vi "LabVIEW_VNA_ESP.vi"() -> ()   [LabVIEW 2020]
uses:
  <vilib>/Analysis/Matrix/Numeric/Conversions/Array To Matrix - RA.vi
  <vilib>/Analysis/Matrix/NI_Matrix.lvlib
panel:
  in  "Entrées pour la fonction Plot":T1={"Chemin du fichiers de mesures (doit contenir le nom du fichier)"=path "", "Type de mesure"="1", "Chemin du fichier parametres (doit contenir le nom du fichier)"=path "", "pas"="", "Coordonnée du point d'arrivée "="", "Coordonnée du point de départ "=""}
  out "Scan 2D mag S12 2":dbl[][](graph)
  out "Scan 2D phase S12 2":dbl[][](graph)
  out "Scan 2D mag S21 2":dbl[][](graph)
  out "Scan 2D phase S21 2":dbl[][](graph)
  out "Rotation mag S21 3":cluster{dbl[], dbl[]}(graph)
  out "Rotation phase S12 2":cluster{dbl[], dbl[]}(graph)
  out "Rotation mag S21 2":cluster{dbl[], dbl[]}(graph)
  out "Rotation phase S21 2":cluster{dbl[], dbl[]}(graph)
  in  "?":bool
  in  "Chemins":cluster{"script python":path, "save path":path}={"script python"=path "C:/Users/Thomas/Documents/Galaad_B/labview/VNA_ESP_10_06_25.py", "save path"=path "C:/Users/Thomas/Documents/Galaad_B/vna_data_test_galaad"}
  in  "IP":T2={"IP VNA"="GPIB0::16::INSTR", "IP ESP Scan 2D"="GPIB0::1::INSTR", "IP ESP Rotation"="GPIB0::2::INSTR"}
  in  "Paramètres de mesures (rotation et balayage)":T3={"Axe"="5", "unité"="2", "coordonnées du point d'arrivé"="10", "coordonnées du point de départ"="0", "pas"="1", "moyennage sur x mesures"="20", "limite basse du balayage en fréquence (GHz)"="110", "limite haute du balayage en fréquence (GHz)"="170", "nombre de points entre les deux limites de fréquences"="201", "IFBW (Hz)"="1000", "band"="WR6.5_Galaad.csa", "sens (aucun effet sur la fonction balayage)"="-to+", "fréquence pour les plots (GHz)"="140", "Nom du fichier"=""}
  in  "Entrées pour la fonction Move":T4={"Axes"="1", "mouvement"="5", "absolu / relatif"="1", "vitesse"="1", "unité"="2", "ESP"=""}
  out "Scan 2D phase S21":dbl[][](graph)
  out "Scan 2D mag S21":dbl[][](graph)
  out "Scan 2D phase S12":dbl[][](graph)
  out "Rotation mag S21":cluster{dbl[], dbl[]}(graph)
  out "Rotation phase S21":cluster{dbl[], dbl[]}(graph)
  out "Rotation phase S12":cluster{dbl[], dbl[]}(graph)
  out "Rotation mag S21":cluster{dbl[], dbl[]}(graph)
  out "Scan 2D mag S12":dbl[][](graph)
  in  "Operation":string(combo)="Balayage_2D_VNA_ESP"
  out "error out":errorcluster caption="sortie d'erreur"
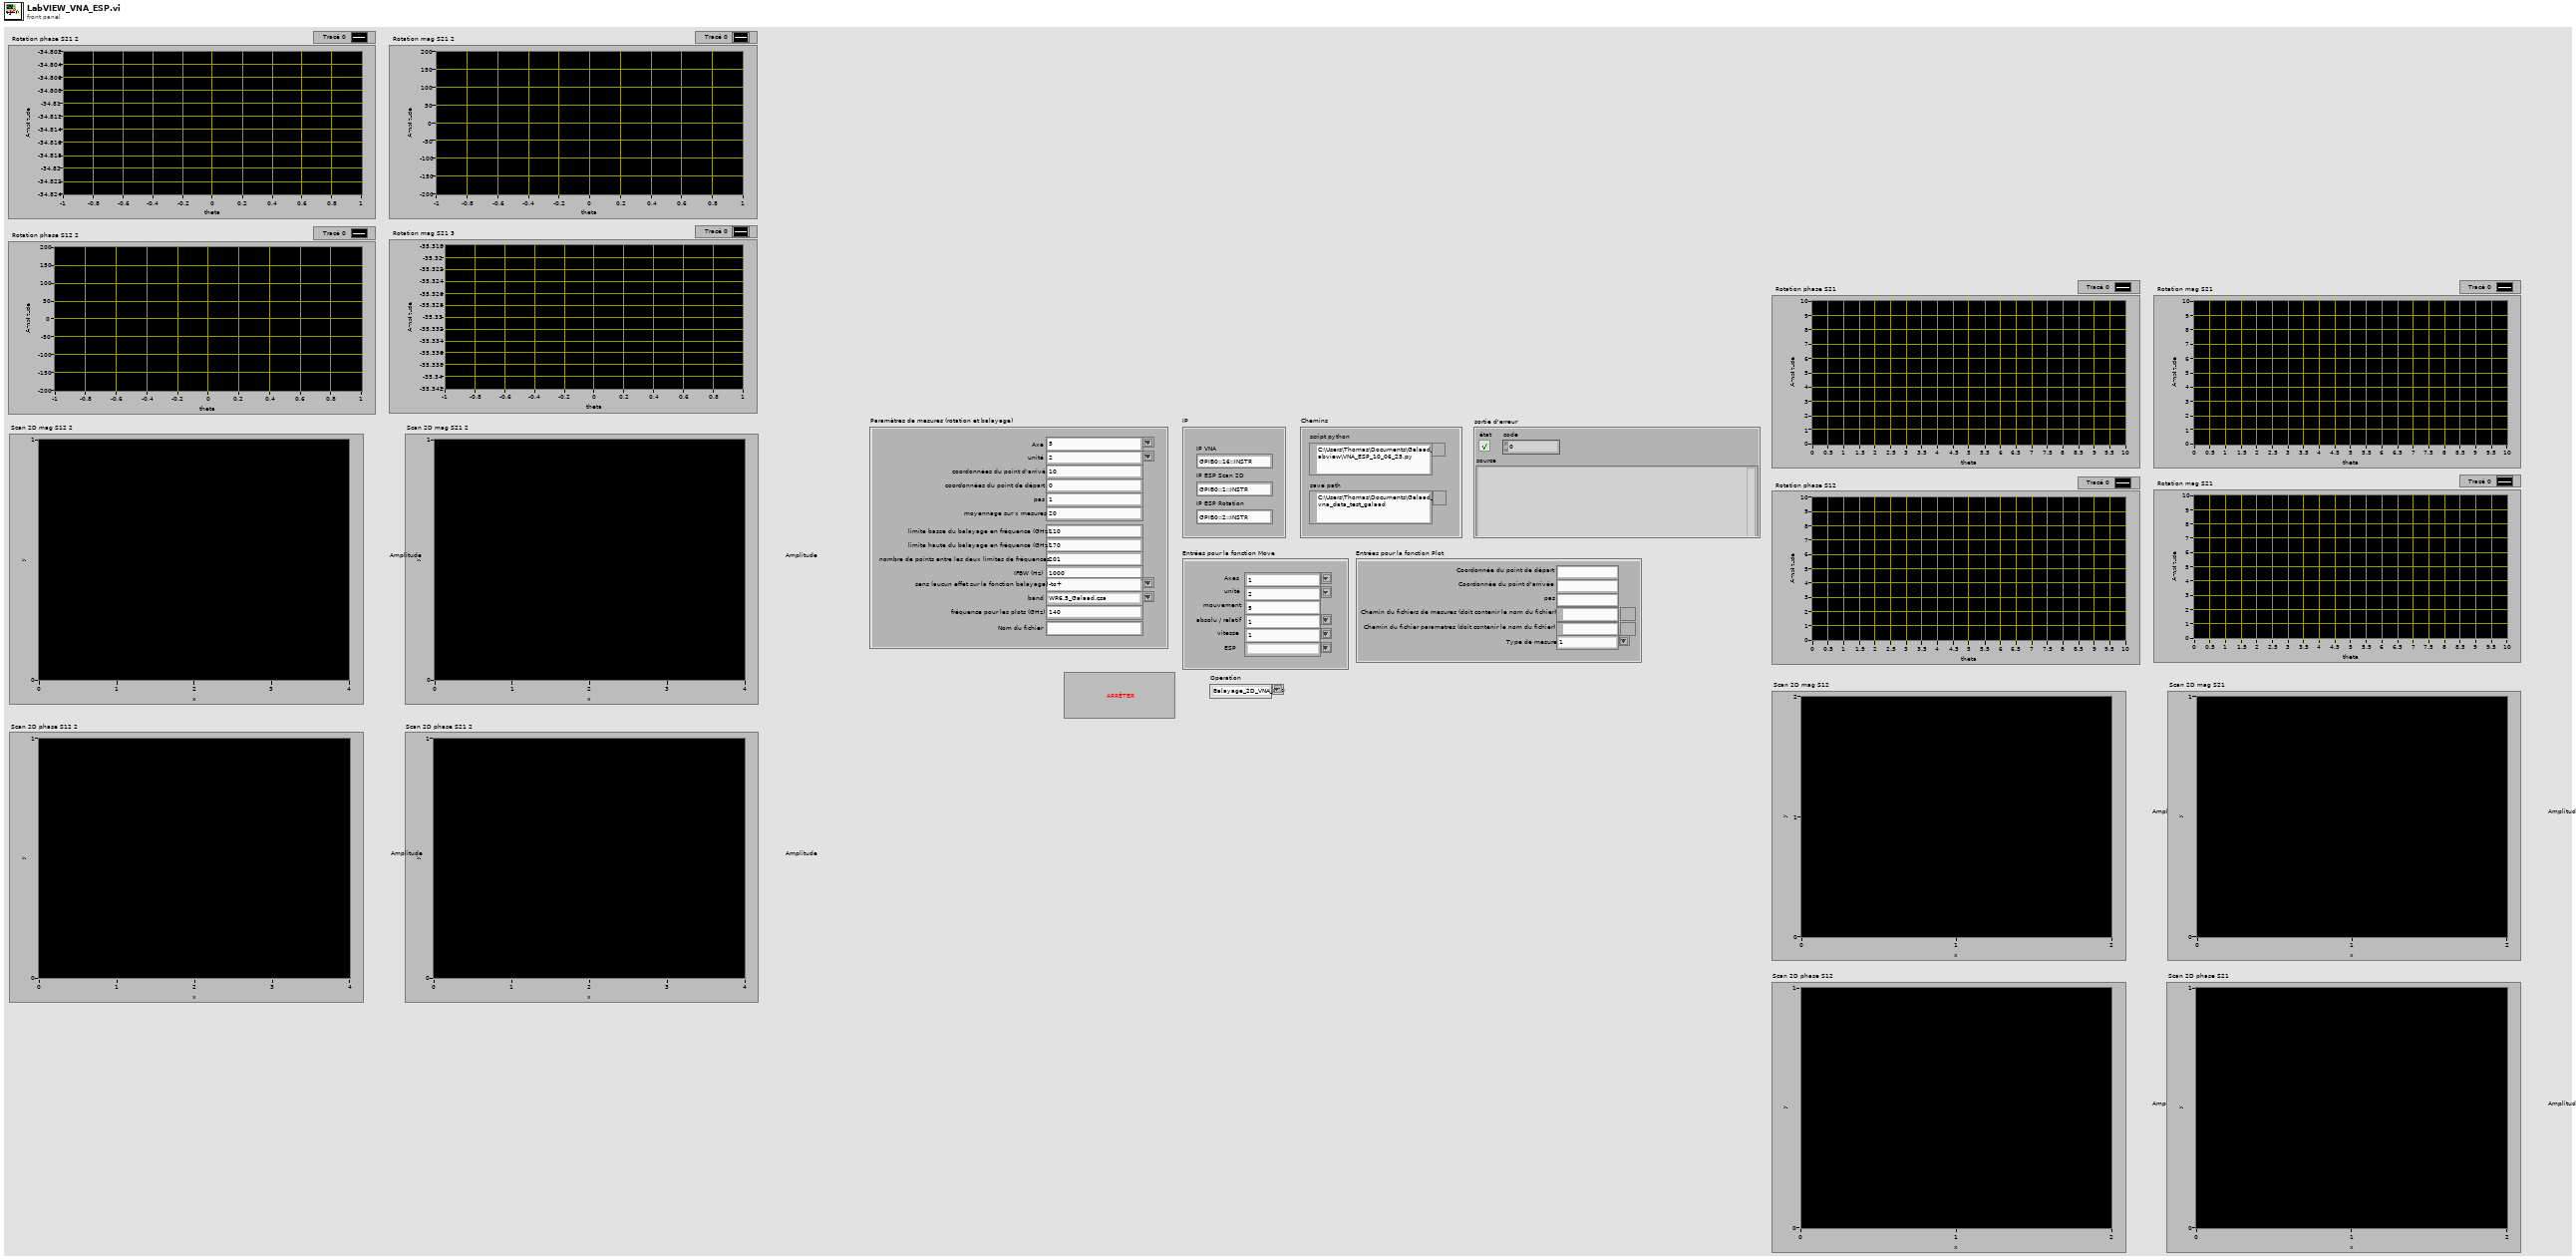
[diagram p1: front panel]
types:
  T1 = cluster{"Chemin du fichiers de mesures (doit contenir le nom du fichier)":path, "Type de mesure":string, "Chemin du fichier parametres (doit contenir le nom du fichier)":path, "pas":string, "Coordonnée du point d'arrivée ":string, "Coordonnée du point de départ ":string}
  T2 = cluster{"IP VNA":string, "IP ESP Scan 2D":string, "IP ESP Rotation":string}
  T3 = cluster{"Axe":string, "unité":string, "coordonnées du point d'arrivé":string, "coordonnées du point de départ":string, "pas":string, "moyennage sur x mesures":string, "limite basse du balayage en fréquence (GHz)":string, "limite haute du balayage en fréquence (GHz)":string, "nombre de points entre les deux limites de fréquences":string, "IFBW (Hz)":string, "band":string, "sens (aucun effet sur la fonction balayage)":string, "fréquence pour les plots (GHz)":string, "Nom du fichier":string}
  T4 = cluster{"Axes":string, "mouvement":string, "absolu / relatif":string, "vitesse":string, "unité":string, "ESP":string}
  T5 = cluster{"Axe":string, "unité":string, "coordonnées du point d'arrivé":string, "coordonnées du point de départ":string, "pas":string, "moyennage sur x mesures":string, "limite basse du balayage en fréquence (GHz)":string, "limite haute du balayage en fréquence (GHz)":string, "nombre de points entre les deux limites de fréquences":string, "IFBW (Hz)":string, "band":string, "IP VNA":string, "IP ESP Scan 2D":string, string, "fréquence pour les plots (GHz)":string, "Nom du fichier":string}
  T6 = cluster{"Axe":string, "unité":string, "coordonnées du point d'arrivé":string, "coordonnées du point de départ":string, "pas":string, "moyennage sur x mesures":string, "limite basse du balayage en fréquence (GHz)":string, "limite haute du balayage en fréquence (GHz)":string, "nombre de points entre les deux limites de fréquences":string, "IFBW (Hz)":string, "band":string, "sens (aucun effet sur la fonction balayage)":string, "fréquence pour les plots (GHz)":string, "IP VNA":string, "IP ESP Rotation":string, string, "Nom du fichier":string}
  T7 = cluster{"Axes":string, "unité":string, "mouvement":string, "absolu / relatif":string, "vitesse":string, "IP ESP Rotation":string}
  T8 = cluster{"Axes":string, "unité":string, "mouvement":string, "absolu / relatif":string, "vitesse":string, "IP ESP Scan 2D":string}
  T9 = typedef "NI_Matrix.lvlib/RealMatrix.ctl" = dbl[][]
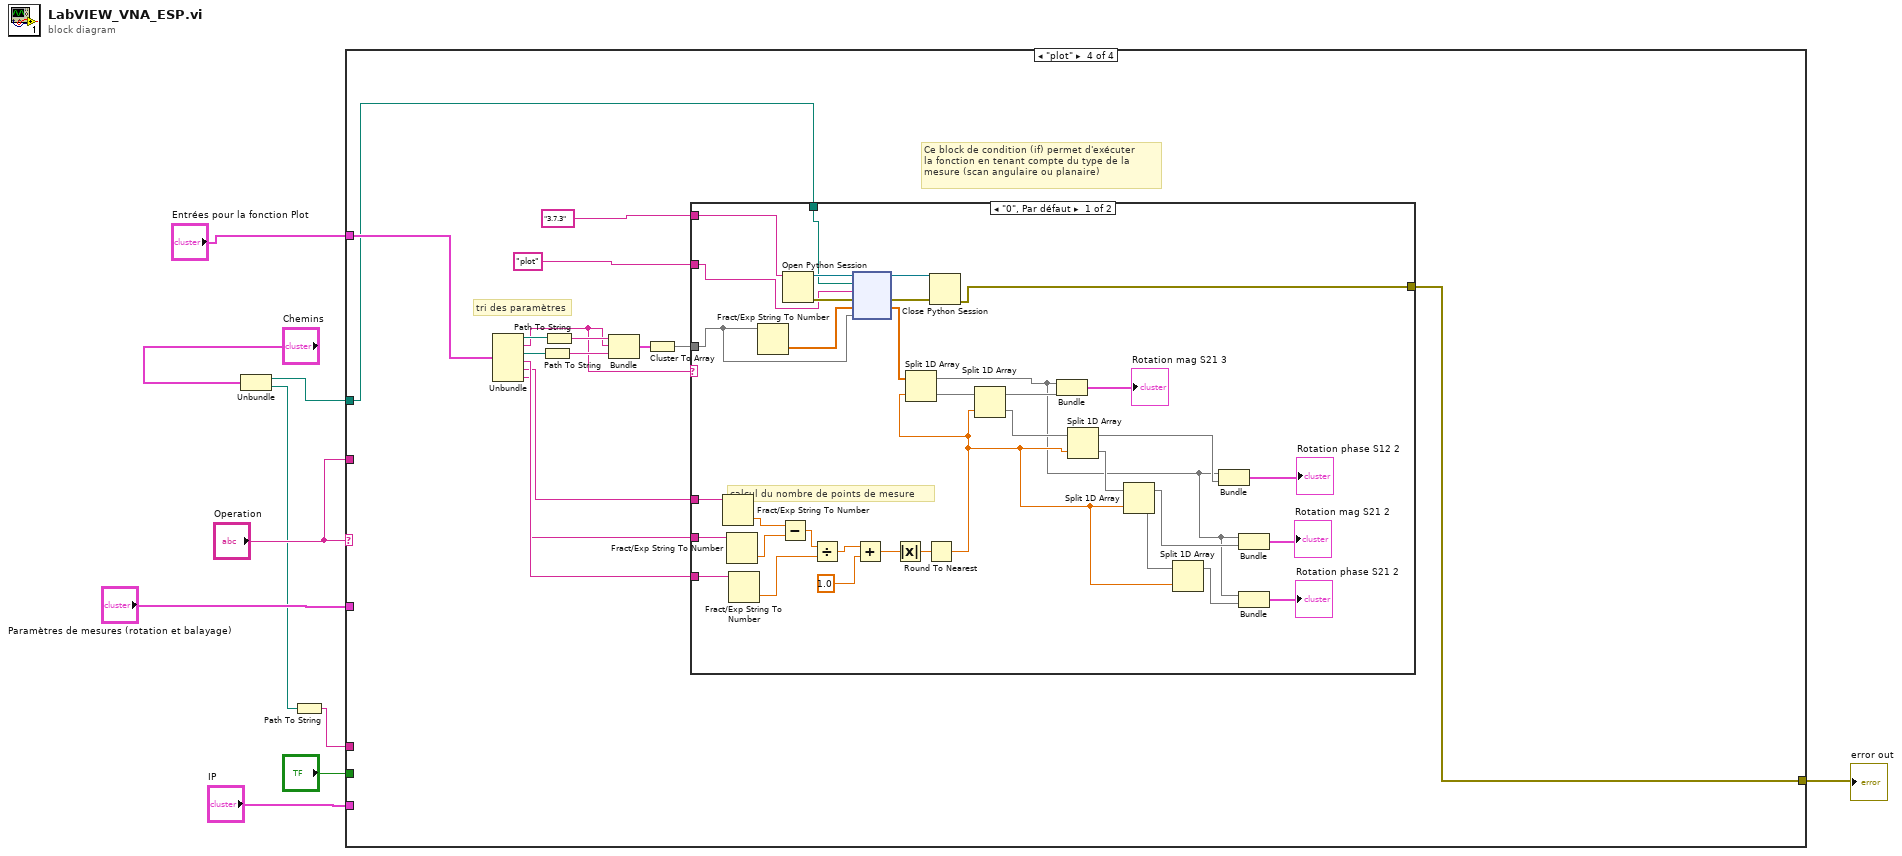
[diagram p0: block diagram]
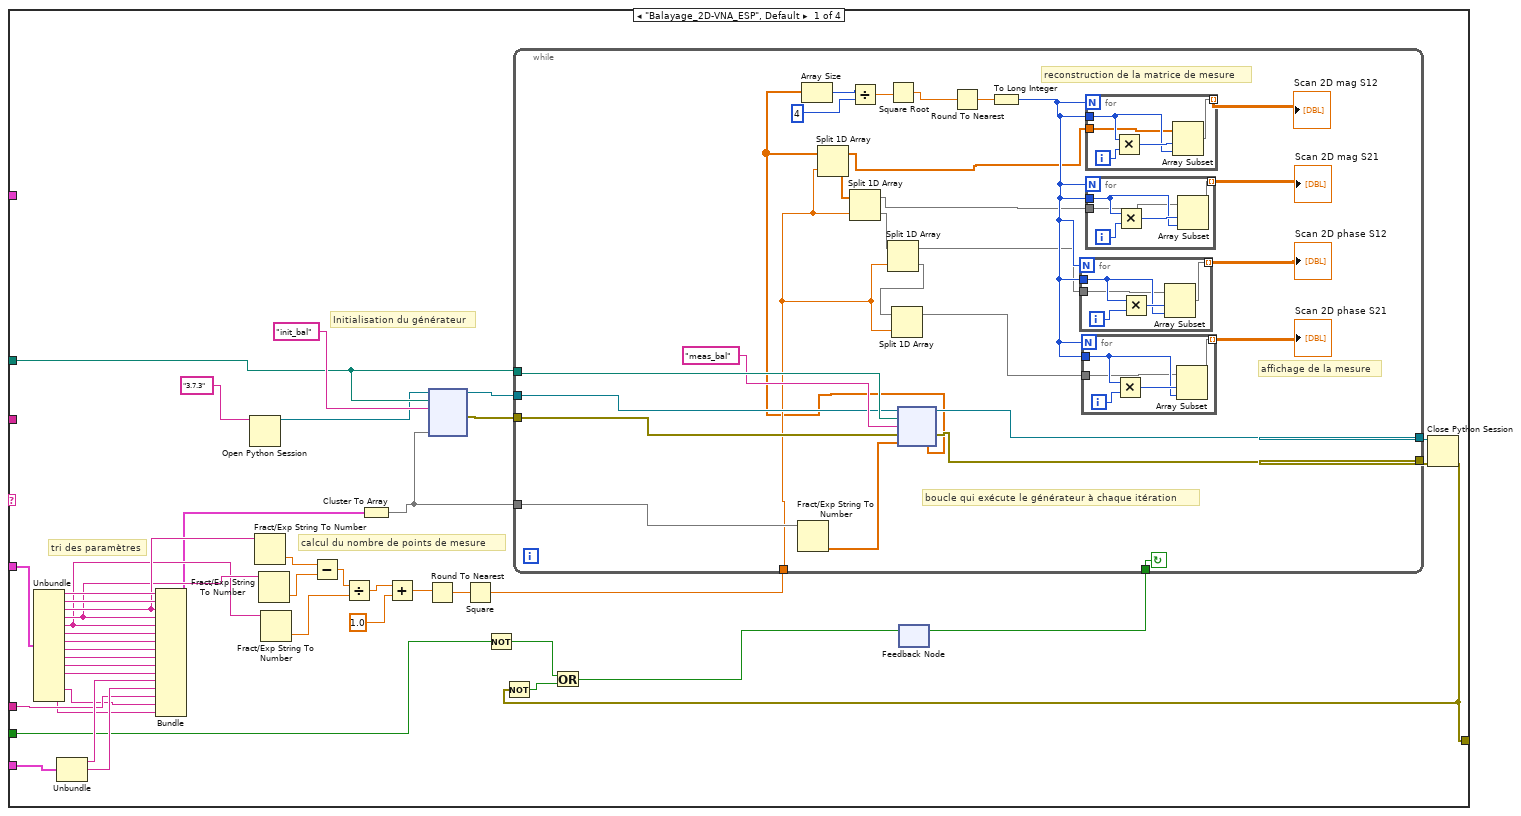
[diagram p2: hidden frame]
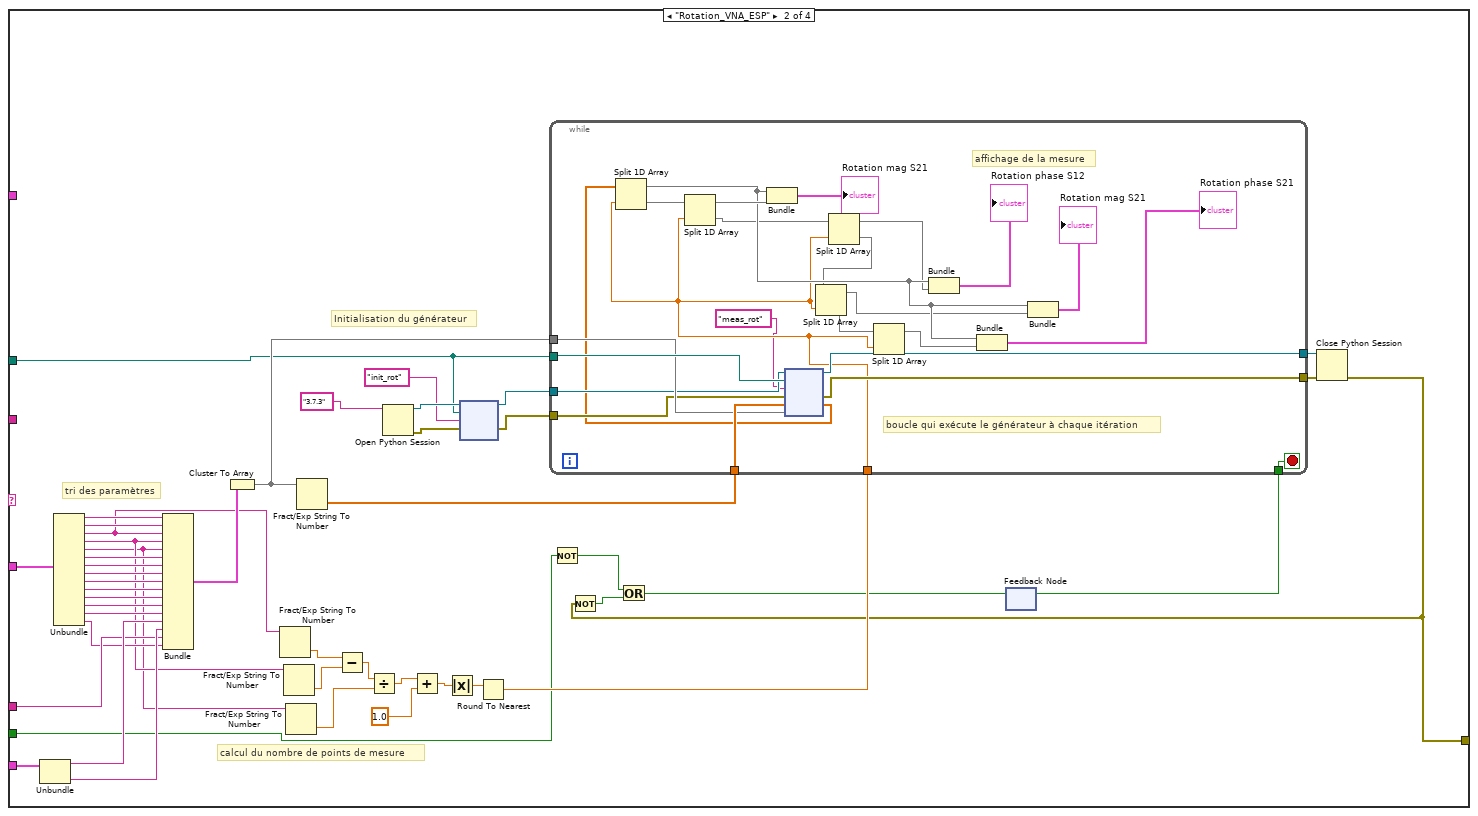
[diagram p3: hidden frame]
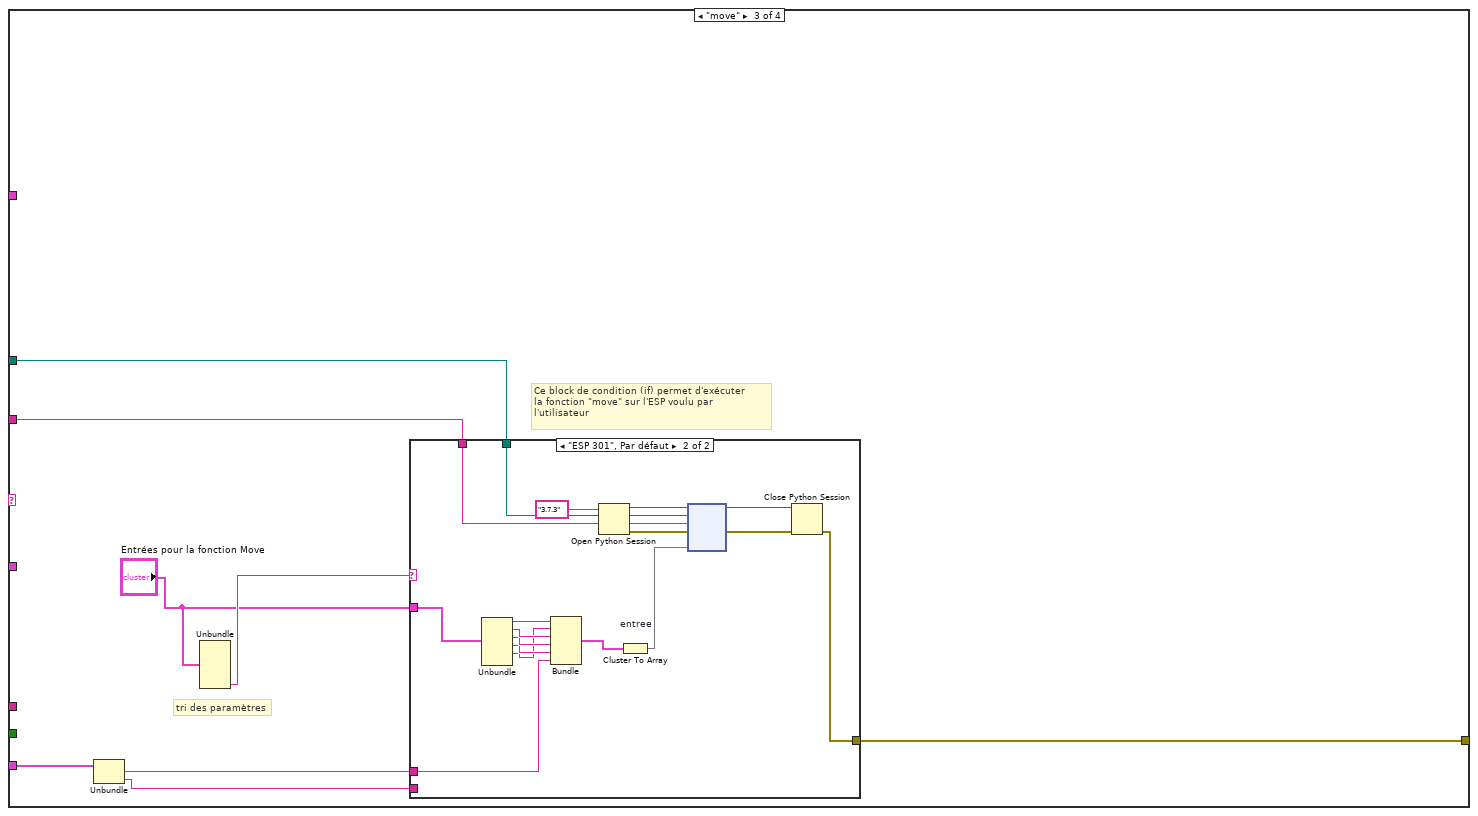
[diagram p4: hidden frame]
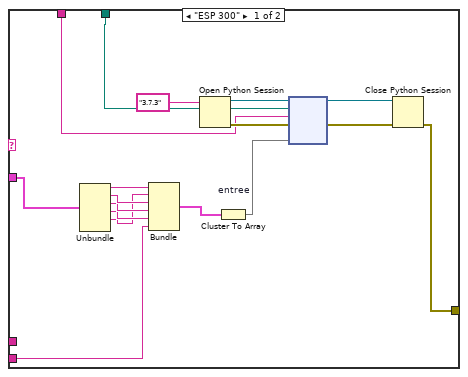
[diagram p5: hidden frame]
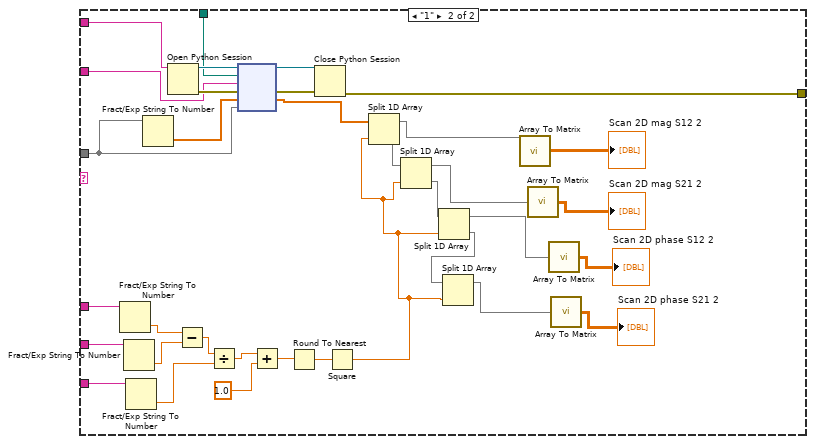
[diagram p6: hidden frame]
diagram:
  n1 = Unbundle("Chemins") -> ("script python"=w4:path, "save path"=w3:path)
  n2 = Path To String(path=w3) -> (string=w10:string)
  n3 = case shown="\"plot\"" "Operation" {
    tunnel: w10 -> [w31 w124 _ _]
    tunnel: "Paramètres de mesures (rotation et balayage)" -> [w34 w139 _ _]
    tunnel: "IP" -> [w46 w138 w177 _]
    tunnel: w4 -> [w19 w114 w174 w215]
    tunnel: [w12 w104 w173 w214] -> w7
    tunnel: "Operation" -> [_ _ w172 _]
    tunnel: "?" -> [w27 w105 _ _]
    tunnel: "Entrées pour la fonction Plot" -> [_ _ _ w216]
    frame "Balayage_2D-VNA_ESP", Default {
      # "tri des paramètres"
      # "calcul du nombre de points de mesure"
      # "Initialisation du générateur"
      n4 = Unbundle(w34) -> ("Axe"=w45:string, "unité"=w44:string, "coordonnées du point d'arrivé"=w37:string, "coordonnées du point de départ"=w36:string, "pas"=w35:string, "moyennage sur x mesures"=w43:string, "limite basse du balayage en fréquence (GHz)"=w42:string, "limite haute du balayage en fréquence (GHz)"=w41:string, "nombre de points entre les deux limites de fréquences"=w40:string, "IFBW (Hz)"=w39:string, "band"=w38:string, "fréquence pour les plots (GHz)"=w30:string, "Nom du fichier"=w29:string)  [unwired: 1 out]
      n5 = Unbundle(w46) -> ("IP VNA"=w33:string, "IP ESP Scan 2D"=w32:string)  [unwired: 1 out]
      n6 = Bundle("Axe"=w45, "unité"=w44, "coordonnées du point d'arrivé"=w37, "coordonnées du point de départ"=w36, "pas"=w35, "moyennage sur x mesures"=w43, "limite basse du balayage en fréquence (GHz)"=w42, "limite haute du balayage en fréquence (GHz)"=w41, "nombre de points entre les deux limites de fréquences"=w40, "IFBW (Hz)"=w39, "band"=w38, "IP VNA"=w33, "IP ESP Scan 2D"=w32, w31, "fréquence pour les plots (GHz)"=w30, "Nom du fichier"=w29) -> (w17:T5)  [unwired: 1 in]
      n7 = Open Python Session(python version="3.7.3") -> (session out=w18:refnum<k35>)  [unwired: 2 in, 1 out]
      n8 = Fract/Exp String To Number(string=w37) -> (number=w51:dbl)  [unwired: 3 in, 1 out]
      n9 = Fract/Exp String To Number(string=w36) -> (number=w52:dbl)  [unwired: 3 in, 1 out]
      n10 = Fract/Exp String To Number(string=w35) -> (number=w53:dbl)  [unwired: 3 in, 1 out]
      n11 = Subtract(x=w51, y=w52) -> (x-y=w48:dbl)
      n12 = Divide(x=w48, y=w53) -> (x/y=w49:dbl)
      n13 = Cluster To Array(cluster=w17) -> (array=w16:string[])
      n14 = Add(x=w49, y=1.0) -> (x+y=w50:dbl)
      n15 = Round To Nearest(number=w50) -> (nearest integer value=w28:dbl)
      n16 = node(w18, w19, "init_bal", w16) -> (w21:refnum<k35>, w15:errorcluster)  [unwired: 4 in, 2 out]
      n17 = Square(x=w28) -> (x^2=w11:dbl)
      n18 = Not(x=w27) -> (.not. x?=w26:bool)
      n19 = feedback #1() -> (w23:bool)  [unwired: 1 in]
      n20 = while {
        tunnel: w23 -> [w81]
        tunnel: w19 -> [w80]
        tunnel: w21 -> [w77]
        tunnel: w16 -> [w76]
        tunnel: w15 -> [w75]
        tunnel: [w74] -> w14
        tunnel: [w73] -> w13
        tunnel: w11 -> [w56]
        stop <- w81 continue-if-true
        # "affichage de la mesure"
        # "reconstruction de la matrice de mesure"
        # "boucle qui exécute le générateur à chaque itération"
        n21 = Fract/Exp String To Number(string=w76) -> (number=w79:dbl[])  [unwired: 3 in, 1 out]
        n22 = node(w77, w80, "meas_bal", w75, w79) -> (w74:refnum<k35>, w73:errorcluster, w54:dbl[])  [unwired: 2 out]
        n23 = Array Size(array=w54) -> (size(s)=w63:i32)
        n24 = Split 1D Array(array=w54, index=w56) -> (first subarray=w55:dbl[], second subarray=w60:dbl[])
        n25 = Divide(x=w63, y=4) -> (x/y=w64:dbl)
        n26 = Split 1D Array(array=w60, index=w56) -> (first subarray=w69:dbl[], second subarray=w59:dbl[])
        n27 = Square Root(x=w64) -> (sqrt(x)=w61:dbl)
        n28 = Split 1D Array(array=w59, index=w56) -> (first subarray=w70:dbl[], second subarray=w58:dbl[])
        n29 = Split 1D Array(array=w58, index=w56) -> (first subarray=w71:dbl[])  [unwired: 1 out]
        n30 = Round To Nearest(number=w61) -> (nearest integer value=w62:dbl)
        n31 = To Long Integer(number=w62) -> (32bit integer=w72:i32)
        n32 = for {
          N: w72 -> [_]
          tunnel: [w91] -> w67 mode=indexing
          tunnel: w72 -> [w88]
          tunnel: w70 -> [w87]
          i -> [w90]
          n33 = Multiply(x=w88, y=w90) -> (x*y=w89:i32)
          n34 = Array Subset(array=w87, index=w89, length=w88) -> (w91:dbl[])
        }
        "Scan 2D phase S12" <- w67
        n35 = for {
          N: w72 -> [_]
          tunnel: [w86] -> w68 mode=indexing
          tunnel: w72 -> [w83]
          tunnel: w71 -> [w82]
          i -> [w85]
          n36 = Multiply(x=w83, y=w85) -> (x*y=w84:i32)
          n37 = Array Subset(array=w82, index=w84, length=w83) -> (w86:dbl[])
        }
        "Scan 2D phase S21" <- w68
        n38 = for {
          N: w72 -> [_]
          tunnel: [w101] -> w65 mode=indexing
          tunnel: w72 -> [w98]
          tunnel: w55 -> [w97]
          i -> [w100]
          n39 = Multiply(x=w98, y=w100) -> (x*y=w99:i32)
          n40 = Array Subset(array=w97, index=w99, length=w98) -> (w101:dbl[])
        }
        "Scan 2D mag S12" <- w65
        n41 = for {
          N: w72 -> [_]
          tunnel: [w96] -> w66 mode=indexing
          tunnel: w72 -> [w93]
          tunnel: w69 -> [w92]
          i -> [w95]
          n42 = Multiply(x=w93, y=w95) -> (x*y=w94:i32)
          n43 = Array Subset(array=w92, index=w94, length=w93) -> (w96:dbl[])
        }
        "Scan 2D mag S21" <- w66
      }
      n44 = Close Python Session(session in=w14, error in=w13) -> (11:w12:errorcluster)
      n45 = Not(x=w12) -> (.not. x?=w25:bool)
      n46 = Or(x=w26, y=w25) -> (x .or. y?=w24:bool)
      n47 = feedback-in #1(w24) -> ()
    }
    frame "Rotation_VNA_ESP" {
      # "calcul du nombre de points de mesure"
      # "Initialisation du générateur"
      # "tri des paramètres"
      n48 = Unbundle(w138) -> ("IP VNA"=w126:string, "IP ESP Rotation"=w125:string)  [unwired: 1 out]
      n49 = Unbundle(w139) -> ("Axe"=w136:string, "unité"=w135:string, "coordonnées du point d'arrivé"=w122:string, "coordonnées du point de départ"=w121:string, "pas"=w120:string, "moyennage sur x mesures"=w134:string, "limite basse du balayage en fréquence (GHz)"=w133:string, "limite haute du balayage en fréquence (GHz)"=w132:string, "nombre de points entre les deux limites de fréquences"=w131:string, "IFBW (Hz)"=w130:string, "band"=w129:string, "sens (aucun effet sur la fonction balayage)"=w128:string, "fréquence pour les plots (GHz)"=w127:string, "Nom du fichier"=w123:string)
      n50 = Bundle("Axe"=w136, "unité"=w135, "coordonnées du point d'arrivé"=w122, "coordonnées du point de départ"=w121, "pas"=w120, "moyennage sur x mesures"=w134, "limite basse du balayage en fréquence (GHz)"=w133, "limite haute du balayage en fréquence (GHz)"=w132, "nombre de points entre les deux limites de fréquences"=w131, "IFBW (Hz)"=w130, "band"=w129, "sens (aucun effet sur la fonction balayage)"=w128, "fréquence pour les plots (GHz)"=w127, "IP VNA"=w126, "IP ESP Rotation"=w125, w124, "Nom du fichier"=w123) -> (w137:T6)  [unwired: 1 in]
      n51 = Cluster To Array(cluster=w137) -> (array=w118:string[])
      n52 = Fract/Exp String To Number(string=w122) -> (number=w143:dbl)  [unwired: 3 in, 1 out]
      n53 = Fract/Exp String To Number(string=w121) -> (number=w144:dbl)  [unwired: 3 in, 1 out]
      n54 = Fract/Exp String To Number(string=w120) -> (number=w145:dbl)  [unwired: 3 in, 1 out]
      n55 = Fract/Exp String To Number(string=w118) -> (number=w119:dbl[])  [unwired: 3 in, 1 out]
      n56 = Subtract(x=w143, y=w144) -> (x-y=w141:dbl)
      n57 = Divide(x=w141, y=w145) -> (x/y=w142:dbl)
      n58 = Open Python Session(python version="3.7.3") -> (session out=w116:refnum<k35>, error out=w115:errorcluster)  [unwired: 2 in]
      n59 = Add(x=w142, y=1.0) -> (x+y=w146:dbl)
      n60 = Absolute Value(x=w146) -> (abs(x)=w147:dbl)
      n61 = node(w116, w114, "init_rot", w115) -> (w112:refnum<k35>, w111:errorcluster)  [unwired: 2 in, 2 out]
      n62 = Round To Nearest(number=w147) -> (nearest integer value=w108:dbl)
      n63 = Not(x=w105) -> (.not. x?=w107:bool)
      n64 = feedback #2() -> (w102:bool)  [unwired: 1 in]
      n65 = while {
        tunnel: w114 -> [w171]
        tunnel: w119 -> [w170]
        tunnel: w118 -> [w169]
        tunnel: w112 -> [w168]
        tunnel: w111 -> [w167]
        tunnel: [w166] -> w110
        tunnel: [w165] -> w109
        tunnel: w108 -> [w151]
        tunnel: w102 -> [w149]
        stop <- w149 stop-if-true
        # "affichage de la mesure"
        # "boucle qui exécute le générateur à chaque itération"
        n66 = node(w168, w171, "meas_rot", w167, w170, w169) -> (w166:refnum<k35>, w165:errorcluster, w150:dbl[])  [unwired: 1 in, 2 out]
        n67 = Split 1D Array(array=w150, index=w151) -> (first subarray=w160:dbl[], second subarray=w164:dbl[])
        n68 = Split 1D Array(array=w164, index=w151) -> (first subarray=w163:dbl[], second subarray=w159:dbl[])
        n69 = Bundle(w160, w163) -> (→"Rotation mag S21":cluster{dbl[], dbl[]})  [unwired: 1 in]
        n70 = Split 1D Array(array=w159, index=w151) -> (first subarray=w158:dbl[], second subarray=w157:dbl[])
        n71 = Split 1D Array(array=w157, index=w151) -> (first subarray=w156:dbl[], second subarray=w155:dbl[])
        n72 = Split 1D Array(array=w155, index=w151) -> (first subarray=w154:dbl[])  [unwired: 1 out]
        n73 = Bundle(w160, w158) -> (→"Rotation phase S12":cluster{dbl[], dbl[]})  [unwired: 1 in]
        n74 = Bundle(w160, w154) -> (→"Rotation phase S21":cluster{dbl[], dbl[]})  [unwired: 1 in]
        n75 = Bundle(w160, w156) -> (→"Rotation mag S21":cluster{dbl[], dbl[]})  [unwired: 1 in]
      }
      n76 = Close Python Session(session in=w110, error in=w109) -> (11:w104:errorcluster)
      n77 = Not(x=w104) -> (.not. x?=w106:bool)
      n78 = Or(x=w107, y=w106) -> (x .or. y?=w103:bool)
      n79 = feedback-in #2(w103) -> ()
    }
    frame "move" {
      # "Ce block de condition (if) permet d'exécuter \nla fonction \"move\" sur l'ESP voulu par \nl'utilisateur"
      # "tri des paramètres"
      n80 = Unbundle(w177) -> ("IP ESP Scan 2D"=w176:string, "IP ESP Rotation"=w175:string)  [unwired: 1 out]
      n81 = Unbundle("Entrées pour la fonction Move") -> ("ESP"=w179:string)  [unwired: 5 out]
      n82 = case shown="\"ESP 301\", Par défaut" w179 {
        tunnel: [w191 w209] -> w173
        tunnel: "Entrées pour la fonction Move" -> [w188 w203]
        tunnel: w176 -> [_ w204]
        tunnel: w175 -> [w186 _]
        tunnel: w174 -> [w185 w208]
        tunnel: w172 -> [w184 w207]
        frame "ESP 300" {
          n83 = Unbundle(w188) -> ("Axes"=w190:string, "mouvement"=w183:string, "absolu / relatif"=w182:string, "vitesse"=w181:string, "unité"=w180:string)  [unwired: 1 out]
          n84 = Bundle("Axes"=w190, "unité"=w180, "mouvement"=w183, "absolu / relatif"=w182, "vitesse"=w181, "IP ESP Rotation"=w186) -> (w189:T7)  [unwired: 1 in]
          n85 = Open Python Session(python version="3.7.3") -> (session out=w195:refnum<k35>, error out=w194:errorcluster)  [unwired: 2 in]
          n86 = Cluster To Array "entree"(cluster=w189) -> (array=w187:string[])
          n87 = node(w195, w185, w184, w194, w187) -> (w196:refnum<k35>, w193:errorcluster)  [unwired: 3 in, 2 out]
          n88 = Close Python Session(session in=w196, error in=w193) -> (11:w191:errorcluster)
        }
        frame "ESP 301", Default {
          n89 = Unbundle(w203) -> ("Axes"=w202:string, "mouvement"=w201:string, "absolu / relatif"=w200:string, "vitesse"=w199:string, "unité"=w198:string)  [unwired: 1 out]
          n90 = Bundle("Axes"=w202, "unité"=w198, "mouvement"=w201, "absolu / relatif"=w200, "vitesse"=w199, "IP ESP Scan 2D"=w204) -> (w206:T8)  [unwired: 1 in]
          n91 = Open Python Session(python version="3.7.3") -> (session out=w212:refnum<k35>, error out=w211:errorcluster)  [unwired: 2 in]
          n92 = Cluster To Array "entree"(cluster=w206) -> (array=w205:string[])
          n93 = node(w212, w208, w207, w211, w205) -> (w213:refnum<k35>, w210:errorcluster)  [unwired: 3 in, 2 out]
          n94 = Close Python Session(session in=w213, error in=w210) -> (11:w209:errorcluster)
        }
      }
    }
    frame "plot" {
      # "tri des paramètres"
      # "Ce block de condition (if) permet d'exécuter \nla fonction en tenant compte du type de la \nmesure (scan angulaire ou planaire)"
      n95 = Unbundle(w216) -> ("Chemin du fichiers de mesures (doit contenir le nom du fichier)"=w227:path, "Type de mesure"=w221:string, "Chemin du fichier parametres (doit contenir le nom du fichier)"=w226:path, "pas"=w219:string, "Coordonnée du point d'arrivée"=w217:string, "Coordonnée du point de départ"=w218:string)
      n96 = Path To String(path=w226) -> (string=w224:string)
      n97 = Path To String(path=w227) -> (string=w225:string)
      n98 = Bundle(w225, "Type de mesure"=w221, w224) -> (w223:cluster{string, "Type de mesure":string, string})  [unwired: 1 in]
      n99 = Cluster To Array(cluster=w223) -> (array=w222:string[])
      n100 = case shown="\"0\", Par défaut" w221 {
        tunnel: [w231 w295] -> w214
        tunnel: w215 -> [w259 w293]
        tunnel: "plot" -> [w258 w292]
        tunnel: w222 -> [w257 w291]
        tunnel: "3.7.3" -> [w256 w277]
        tunnel: w219 -> [w235 w268]
        tunnel: w218 -> [w234 w269]
        tunnel: w217 -> [w233 w270]
        frame "0", Default {
          # "calcul du nombre de points de mesure"
          n101 = Fract/Exp String To Number(string=w233) -> (number=w238:dbl)  [unwired: 3 in, 1 out]
          n102 = Fract/Exp String To Number(string=w234) -> (number=w239:dbl)  [unwired: 3 in, 1 out]
          n103 = Fract/Exp String To Number(string=w235) -> (number=w240:dbl)  [unwired: 3 in, 1 out]
          n104 = Fract/Exp String To Number(string=w257) -> (number=w260:dbl[])  [unwired: 3 in, 1 out]
          n105 = Subtract(x=w238, y=w239) -> (x-y=w236:dbl)
          n106 = Open Python Session(python version=w256) -> (session out=w264:refnum<k35>, error out=w261:errorcluster)  [unwired: 2 in]
          n107 = Divide(x=w236, y=w240) -> (x/y=w237:dbl)
          n108 = node(w264, w259, w258, w261, w260, w257) -> (w263:refnum<k35>, w262:errorcluster, w243:dbl[])  [unwired: 1 in, 2 out]
          n109 = Add(x=w237, y=1.0) -> (x+y=w242:dbl)
          n110 = Absolute Value(x=w242) -> (abs(x)=w241:dbl)
          n111 = Round To Nearest(number=w241) -> (nearest integer value=w230:dbl)
          n112 = Split 1D Array(array=w243, index=w230) -> (first subarray=w229:dbl[], second subarray=w244:dbl[])
          n113 = Close Python Session(session in=w263, error in=w262) -> (11:w231:errorcluster)
          n114 = Split 1D Array(array=w244, index=w230) -> (first subarray=w245:dbl[], second subarray=w248:dbl[])
          n115 = Bundle(w229, w245) -> (→"Rotation mag S21 3":cluster{dbl[], dbl[]})  [unwired: 1 in]
          n116 = Split 1D Array(array=w248, index=w230) -> (first subarray=w249:dbl[], second subarray=w250:dbl[])
          n117 = Split 1D Array(array=w250, index=w230) -> (first subarray=w251:dbl[], second subarray=w252:dbl[])
          n118 = Split 1D Array(array=w252, index=w230) -> (first subarray=w253:dbl[])  [unwired: 1 out]
          n119 = Bundle(w229, w249) -> (→"Rotation phase S12 2":cluster{dbl[], dbl[]})  [unwired: 1 in]
          n120 = Bundle(w229, w251) -> (→"Rotation mag S21 2":cluster{dbl[], dbl[]})  [unwired: 1 in]
          n121 = Bundle(w229, w253) -> (→"Rotation phase S21 2":cluster{dbl[], dbl[]})  [unwired: 1 in]
        }
        frame "1" {
          n122 = Fract/Exp String To Number(string=w270) -> (number=w274:dbl)  [unwired: 3 in, 1 out]
          n123 = Fract/Exp String To Number(string=w269) -> (number=w275:dbl)  [unwired: 3 in, 1 out]
          n124 = Fract/Exp String To Number(string=w268) -> (number=w276:dbl)  [unwired: 3 in, 1 out]
          n125 = Fract/Exp String To Number(string=w291) -> (number=w290:dbl[])  [unwired: 3 in, 1 out]
          n126 = Open Python Session(python version=w277) -> (session out=w298:refnum<k35>, error out=w294:errorcluster)  [unwired: 2 in]
          n127 = Subtract(x=w274, y=w275) -> (x-y=w272:dbl)
          n128 = Divide(x=w272, y=w276) -> (x/y=w273:dbl)
          n129 = node(w298, w293, w292, w294, w290, w291) -> (w297:refnum<k35>, w296:errorcluster, w278:dbl[])  [unwired: 1 in, 2 out]
          n130 = Add(x=w273, y=1.0) -> (x+y=w266:dbl)
          n131 = Round To Nearest(number=w266) -> (nearest integer value=w267:dbl)
          n132 = Close Python Session(session in=w297, error in=w296) -> (11:w295:errorcluster)
          n133 = Square(x=w267) -> (x^2=w265:dbl)
          n134 = Split 1D Array(array=w278, index=w265) -> (first subarray=w287:dbl[], second subarray=w285:dbl[])
          n135 = Split 1D Array(array=w285, index=w265) -> (first subarray=w284:dbl[], second subarray=w283:dbl[])
          n136 = Split 1D Array(array=w283, index=w265) -> (first subarray=w282:dbl[], second subarray=w281:dbl[])
          n137 = Split 1D Array(array=w281, index=w265) -> (first subarray=w280:dbl[])  [unwired: 1 out]
          n138 = call-poly <vilib>:"Array To Matrix.vi"("Real 1D Array"=w287) -> ("Real Matrix (Column Vector)"=→"Scan 2D mag S12 2":T9)
          n139 = call-poly <vilib>:"Array To Matrix.vi"("Real 1D Array"=w284) -> ("Real Matrix (Column Vector)"=→"Scan 2D mag S21 2":T9)
          n140 = call-poly <vilib>:"Array To Matrix.vi"("Real 1D Array"=w282) -> ("Real Matrix (Column Vector)"=→"Scan 2D phase S12 2":T9)
          n141 = call-poly <vilib>:"Array To Matrix.vi"("Real 1D Array"=w280) -> ("Real Matrix (Column Vector)"=→"Scan 2D phase S21 2":T9)
        }
      }
    }
  }
  "error out" <- w7
